vi "Calibrator Sub.vi"(0 "Connection ID in":refnum<k5>, 5 "Sensor Array":T2, 9 "history length":u16=100 min=1, 11 "Index":u32[](array[numeric])) -> (4 "Sensor Data":T4 {"Sensor array"."scaled" format="%.2f"; "Sensor array"."voltage" format="%.4f"; "Time" format="%<%I:%M:%S%2u %p\n%m/%d/%Y>T"}, 12 "Index":u32, 15 "Data Display":T1 {"average data rate (Hz)" format="%.2f"; "Min Range" format="%.3f"; "Max Range" format="%.3f"; "Mean (Volts)" format="%.5f"; "Mean (scaled)" format="%.2f"})   [LabVIEW 2010]
uses:
  global scale array.vi
  DAQ configuration/Sensor buffer command.ctl
  DAQ configuration/sensor cluster.ctl
  TCP DAQ/Sensor data.ctl
  DAQ configuration/channel identifier.ctl
  DAQ configuration/Sensor array.ctl
  calibrator graph.ctl
panel:
  # "V"
  # "V"
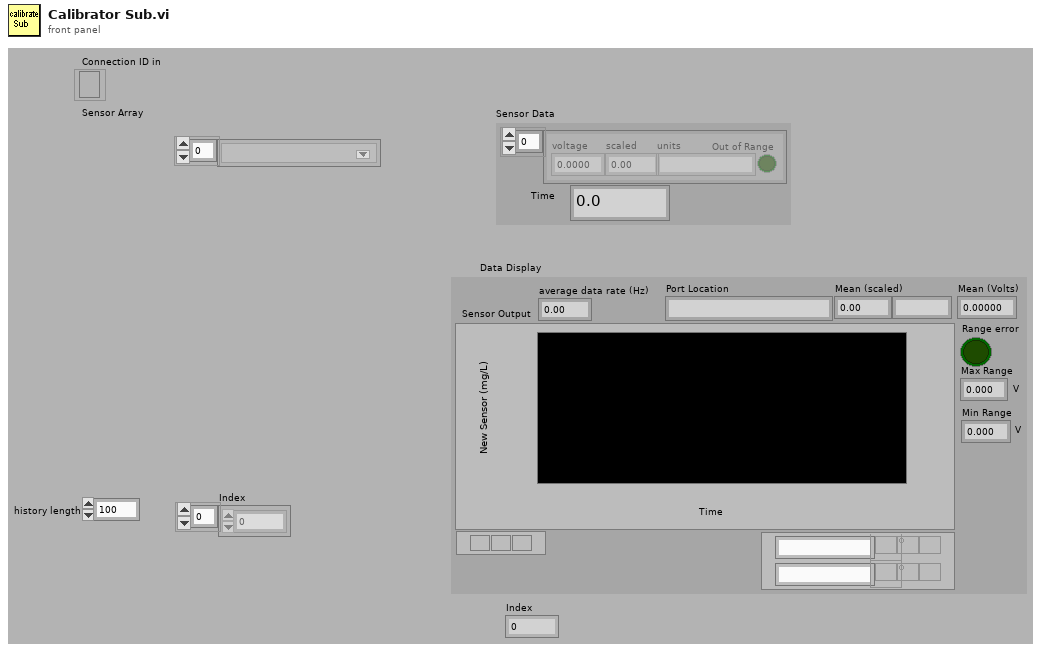
[diagram p1: front panel]
types:
  T1 = typedef "calibrator graph.ctl" = cluster{"Range error":bool, "Mean (scaled)":dbl, "Mean (Volts)":dbl, "Max Range":dbl, "Min Range":dbl, "units":string, "Sensor Output":cluster{dbl[], dbl[]}[], "Port Location":string, "average data rate (Hz)":dbl}
  T2 = typedef "Sensor array.ctl" = T3[]
  T3 = typedef "channel identifier.ctl" = u16
  T4 = typedef "Sensor data.ctl" = cluster{" Sensor array":T5[], "Time":dbl}
  T5 = typedef "sensor cluster.ctl" = cluster{"voltage":sgl, "scaled":sgl, "units":string, "Out of Range":bool}
  T6 = typedef "Sensor buffer command.ctl" = enum16{"read average", "read recent", "read all", "write", "configure", "clear"}
  T7 = typedef "calib array.ctl" = T8[]
  T8 = typedef "conversion.ctl" = cluster{"conversion matrix":sgl[][], "units":string, "name":string, "scale type":T9, "offset (volts)":dbl, "second channel":i8, "correspondence table":T10, "offset (physical units)":dbl, "pH scale":T11, "D.O.":T12}
  T9 = typedef "scale type.ctl" = enum16{"Volts", "Polynomial", "Correspondence Table", "pH", "Dissolved Oxygen", "Quadratic"}
  T10 = typedef "correspondence table.ctl" = cluster{"physical units":dbl, "volts":dbl}[]
  T11 = typedef "pH scale.ctl" = cluster{"Buffers":cluster{"Buffer":dbl, "Calibrated":bool, "V/T":dbl}[], "Temperature":dbl}
  T12 = typedef "DO scale.ctl" = cluster{"Temperature":dbl, "K":dbl, "barometric pressure":dbl}
  T13 = typedef "data status.ctl" = enum16{"Okay", "Sensor Range error", "Server error"}
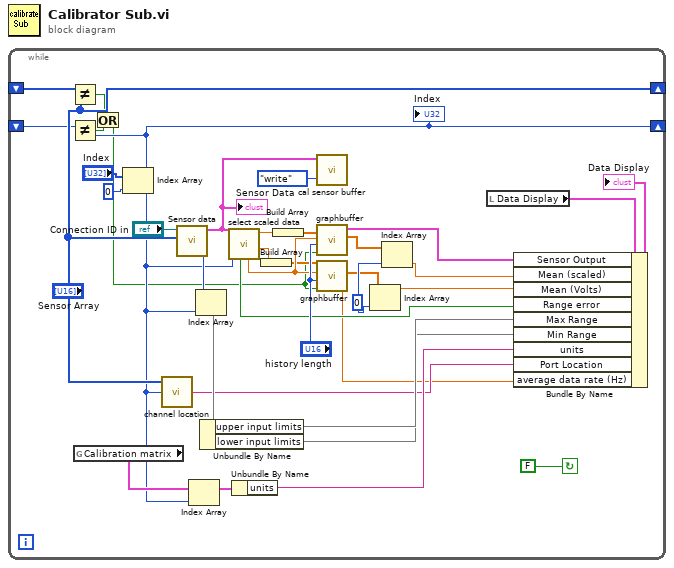
[diagram p0: block diagram]
diagram:
  n1 = while {
    shift-left: _ -> [w24]
    shift-right: [w5] -> _
    shift-left: _ -> [w27]
    shift-right: ["Sensor Array"] -> _
    stop <- FALSE continue-if-true
    w34 = 0 ("Index")
    n2 = Not Equal?(x=w27, y="Sensor Array") -> (x != y?=w23:bool)
    n3 = global read "global scale array.vi" "Calibration matrix"() -> (w17:T7)
    n4 = Index Array(array="Index", index=0 ("Index")) -> (element=w5:u32)
    "Index" <- w5
    n5 = Not Equal?(x=w24, y=w5) -> (x != y?=w22:bool)
    n6 = Or(x=w23, y=w22) -> (x .or. y?=w3:bool)
    n7 = call "channel location.vi"("Index"=w5, "Sensor Array"="Sensor Array") -> ("Port Location"=w6:string)  [unwired: 1 in]
    n8 = call "Sensor data.vi"("Sensor Array"="Sensor Array", "Connection ID in"="Connection ID in") -> ("Data Status"=w20:T13, "Sensor Data"=w2:T4)  [unwired: 2 in, 6 out]
    "Sensor Data" <- w2
    n9 = Index Array(array=w17, index=w5) -> (element=w16:T8)
    n10 = Index Array(array=w20, index=w5) -> (element=w19)
    n11 = Unbundle By Name(w19) -> ("upper input limits"=w9, "lower input limits"=w8)
    n12 = call "select scaled data.vi"("Sensor index"=w5, "Sensor Data"=w2) -> ("voltage"=w30:sgl, "scaled"=w37:sgl, "Time"=w31:dbl, "Out of Range"=w10:bool)  [unwired: 3 in, 1 out]
    n13 = Unbundle By Name(w16) -> ("units"=w7:string)
    n14 = Build Array(w30) -> (w29:sgl[])
    n15 = Build Array(w37) -> (w36:sgl[])
    n16 = call "cal sensor buffer.vi"("command"=Sensor_buffer_command."write", "Sensor Data"=w2) -> ()  [unwired: 3 in, 3 out]
    n17 = call "graphbuffer.vi"("Reset"=w3, "history length"="history length", "Time"=w31, "data"=w36) -> ("Mean"=w28:dbl[], "Multiplot graph data"=w13:cluster{dbl[], dbl[]}[])  [unwired: 5 in, 1 out]
    n18 = call "graphbuffer.vi"("Reset"=w3, "history length"="history length", "Time"=w31, "data"=w29) -> ("data rate (Hz)"=w4:dbl, "Mean"=w32:dbl[])  [unwired: 5 in, 1 out]
    n19 = Index Array(array=w32, index=w34) -> (element=w11:dbl)
    n20 = Index Array(array=w28, index=w34) -> (element=w12:dbl)
    n21 = local read "Data Display"() -> (w14:T1)
    n22 = Bundle By Name(cluster=w14, "Sensor Output"=w13, "Mean (scaled)"=w12, "Mean (Volts)"=w11, "Range error"=w10, "Max Range"=w9, "Min Range"=w8, "units"=w7, "Port Location"=w6, "average data rate (Hz)"=w4) -> (→"Data Display":T1)
  }
